vi "Parameter Setup( Single Functional).vi"() -> (2 "Run?":bool, 3 "Position(out)":i32 min=1 max=32 step=1, 5 "Channel(s) (out)":u16(ring) items=["1+2", "1", "2", "3"])   [LabVIEW 2024]
panel:
  in  "Channel(s)":u16(ring) items=["1+2", "1", "2", "3"]
  in  "Position":i32=1 min=1 max=32 step=1
  in  "Enter":bool
  # "Please Enter Position Number"
  # "Legend:\nChannel(s): Channels used on\nFrequency Counter (1+2 = 16 and 16)"
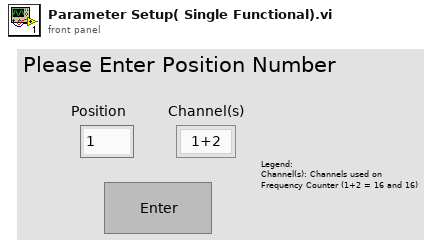
[diagram p1: front panel]
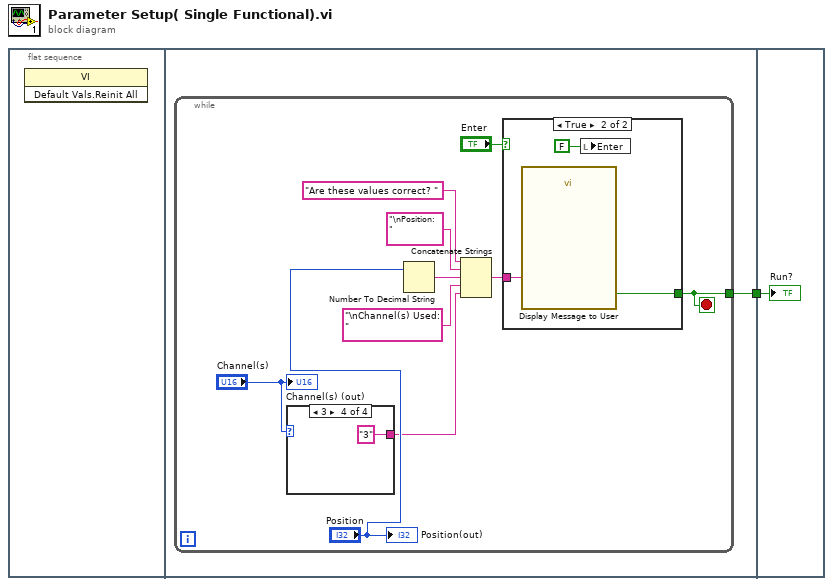
[diagram p0: block diagram]
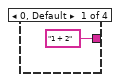
[diagram p2: hidden frame]
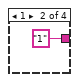
[diagram p3: hidden frame]
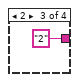
[diagram p4: hidden frame]
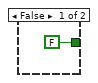
[diagram p5: hidden frame]
diagram:
  n1 = flat-sequence {
    tunnel: [w2] -> w1
    tunnel: w1 -> [w21]
    frame #0 {
      n2 = invoke class="VI" method="Default Vals.Reinit All"() -> ()  [unwired: 3 in, 3 out]
    }
    frame #1 {
      n3 = while {
        tunnel: [w6] -> w2
        stop <- w6 stop-if-true
        n4 = case shown="3" "Channel(s)" {
          tunnel: ["1 + 2" "1" "2" "3"] -> w3
          frame 0, Default {
          }
          frame 1 {
          }
          frame 2 {
          }
          frame 3 {
          }
        }
        n5 = Number To Decimal String(number="Position") -> (decimal integer string=w7:string)  [unwired: 1 in]
        n6 = Concatenate Strings("Are these values correct? ", "\nPosition: " ("string"), w7, "\nChannel(s) Used: " ("string"), w3) -> (w9:string)
        n7 = case shown="True" "Enter" {
          tunnel: [FALSE w19] -> w6
          tunnel: w9 -> [_ w18]
          frame False {
          }
          frame True {
            n8 = call "Display Message to User"("Message"=w18) -> ("Yes"=w19:bool)  [unwired: 9 in, 1 out]
            n9 = local write "Enter"(FALSE ("Enter")) -> ()
          }
        }
        "Position(out)" <- "Position"
        "Channel(s) (out)" <- "Channel(s)"
      }
    }
    frame #2 {
      "Run?" <- w21
    }
  }
